vi "TypeToColor.vi"(11 "type":T1) -> (2 "ItemSyms":i32, 3 "Color":u32(colorbox))   [LabVIEW 2020, in "BlueVariantView.lvlib"]
uses:
  BlueVariantView.lvlib
  <vilib>/Utility/Data Type/Type Definitions/Data Type.ctl
  Symbol.ctl
  <vilib>/Utility/Data Type/NI_Data Type.lvlib
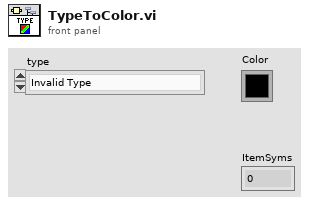
[diagram p1: front panel]
types:
  T1 = typedef "NI_Data Type.lvlib/Data Type.ctl" = enum8{"Invalid Type", "Void", "I8", "I16", "I32", "I64", "U8", "U16", "U32", "U64", "Single Float", "Double Float", "Extended Float", "Single Complex", "Double Complex", "Extended Complex", "Enum U8", "Enum U16", "Enum U32", "Enum U64", "Single Float With Unit", "Double Float With Unit", "Extended Float With Unit", "Single Complex with Unit", "Double Complex with Unit", "Extended Complex with Unit", "Boolean", "String", "Path", "Picture", "Tag", "Array", "Cluster", "Variant", "LV Variant", "Waveform", "Timestamp", "Digital Waveform", "Digital Data", "ExpressData", "Refnum", "External Data", "VI", "Poly VI", "LabVIEW Class Instance", "Fixed Point", "Set Collection", "Map Collection"}
  T2 = typedef "BlueVariantView.lvlib/Symbol.ctl" = enum16{"None", "Cluster-brown", "Cluster-yellow", "Cluster-black", "Cluster-pink", "Array", "Float", "Int", "Bool", "String", "Enum", "Object", "Map", "Set", "Refnum", "Variant", "Path", "Picture", "Waveform", "Timestamp", "Digital Waveform", "Fixed Point"}
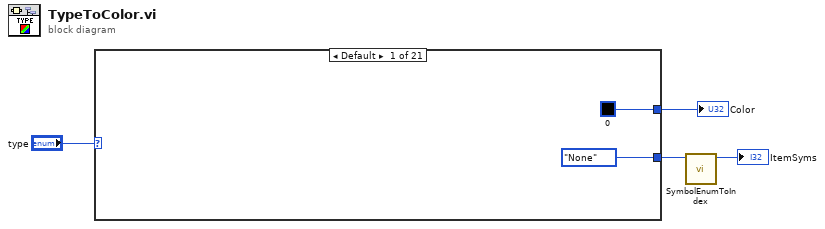
[diagram p0: block diagram]
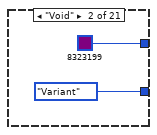
[diagram p2: hidden frame]
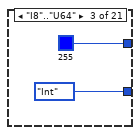
[diagram p3: hidden frame]
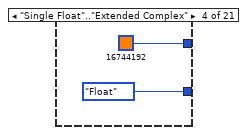
[diagram p4: hidden frame]
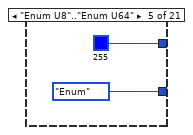
[diagram p5: hidden frame]
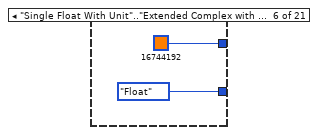
[diagram p6: hidden frame]
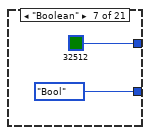
[diagram p7: hidden frame]
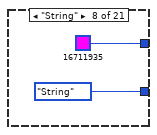
[diagram p8: hidden frame]
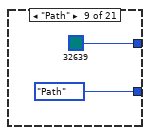
[diagram p9: hidden frame]
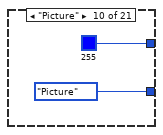
[diagram p10: hidden frame]
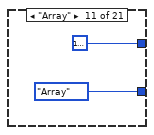
[diagram p11: hidden frame]
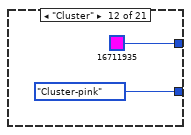
[diagram p12: hidden frame]
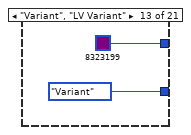
[diagram p13: hidden frame]
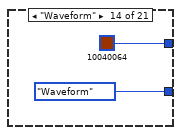
[diagram p14: hidden frame]
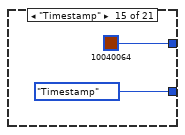
[diagram p15: hidden frame]
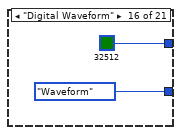
[diagram p16: hidden frame]
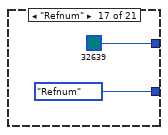
[diagram p17: hidden frame]
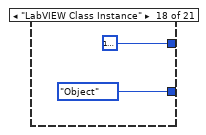
[diagram p18: hidden frame]
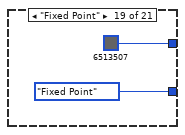
[diagram p19: hidden frame]
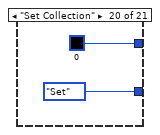
[diagram p20: hidden frame]
diagram:
  n1 = case shown="Default" "type" {
    tunnel: [u32 0 u32 8323199 u32 255 u32 16744192 u32 255 u32 16744192 u32 32512 u32 16711935 u32 32639 u32 255 u32 16777222 u32 16711935 u32 8323199 u32 10040064 u32 10040064 u32 32512 u32 32639 u32 16777222 u32 6513507 u32 0 u32 0] -> w3
    tunnel: [Symbol."None" ("Symbol") Symbol."Variant" ("Symbol") Symbol."Int" ("Symbol") Symbol."Float" ("Symbol") Symbol."Enum" ("Symbol") Symbol."Float" ("Symbol") Symbol."Bool" ("Symbol") Symbol."String" ("Symbol") Symbol."Path" ("Symbol") Symbol."Picture" ("Symbol") Symbol."Array" ("Symbol") Symbol."Cluster-pink" ("Symbol") Symbol."Variant" ("Symbol") Symbol."Waveform" ("Symbol") Symbol."Timestamp" ("Symbol") Symbol."Waveform" ("Symbol") Symbol."Refnum" ("Symbol") Symbol."Object" ("Symbol") Symbol."Fixed Point" ("Symbol") Symbol."Set" ("Symbol") Symbol."Map" ("Symbol")] -> w2
    frame Default {
    }
    frame "Void" {
    }
    frame "I8".."U64" {
    }
    frame "Single Float".."Extended Complex" {
    }
    frame "Enum U8".."Enum U64" {
    }
    frame "Single Float With Unit".."Extended Complex with Unit" {
    }
    frame "Boolean" {
    }
    frame "String" {
    }
    frame "Path" {
    }
    frame "Picture" {
    }
    frame "Array" {
    }
    frame "Cluster" {
    }
    frame "Variant", "LV Variant" {
    }
    frame "Waveform" {
    }
    frame "Timestamp" {
    }
    frame "Digital Waveform" {
    }
    frame "Refnum" {
    }
    frame "LabVIEW Class Instance" {
    }
    frame "Fixed Point" {
    }
    frame "Set Collection" {
    }
    frame "Map Collection" {
    }
  }
  "Color" <- w3
  n2 = call "SymbolEnumToIndex.vi"("symbol enum"=w2) -> ("ItemSyms"=→"ItemSyms":i32)  [unwired: 10 in]
